vi "Get Boundary and Descriptions.vi"(0 "Image In":T1, 1 "Number of iterations":i32=1, 2 "Out":T1, 3 "In":T1, 5 "Mask In":T1, 9 "Submask":T1, 11 "error in (no error)":errorcluster, 12 "ConvexHull":bool) -> (4 "Boundaries":cluster{cluster{i32, i32}[]}[](array[cluster]), 6 "Reporter":T2(array[cluster]), 10 "Object Descriptions":T3(array[cluster]), 15 "error out":errorcluster)   [LabVIEW 2012, in "Visual Analyser.lvlib"]
uses:
  Visual Analyser.lvlib
  <vilib>/vision/Image Controls.llb/IMAQ Image.ctl
  <vilib>/vision/NI_Vision_Development_Module.lvlib
panel:
  in  "WholeBG %":sgl
  out "#particles":i32
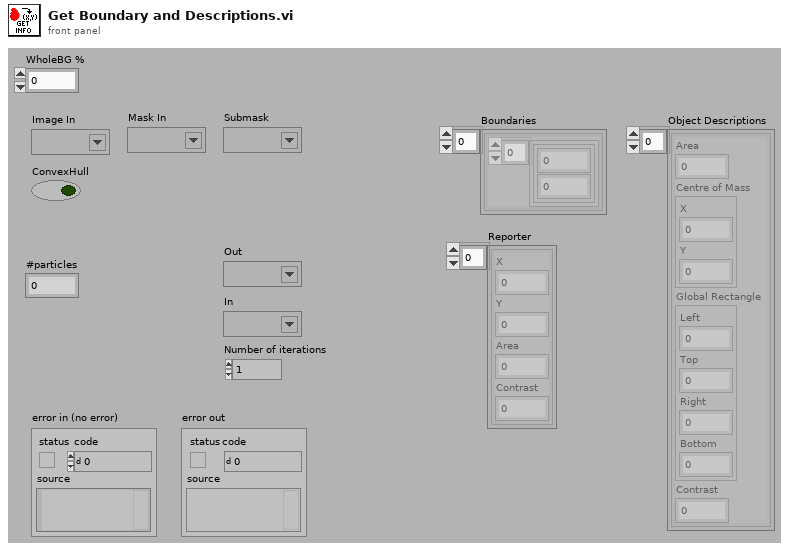
[diagram p1: front panel]
types:
  T1 = typedef "IMAQ Image.ctl" = refnum<image>
  T2 = cluster{"X":dbl, "Y":dbl, "Area":dbl, "Contrast":dbl}[]
  T3 = cluster{"Area":dbl, "Centre of Mass":cluster{"X":dbl, "Y":dbl}, "Global Rectangle":cluster{"Left":dbl, "Top":dbl, "Right":dbl, "Bottom":dbl}, "Contrast":dbl}[]
  T4 = typedef "Particle Parameters" = i32
  T5 = typedef "ROI Descriptor" = cluster{"Global Rectangle":i32[], "Contours":cluster{"ID":enum32{"External", "Internal"}, "Type":u32, "Coordinates":i32[]}[]}
  T6 = enum32{"AutoM", "Close", "Dilate", "Erode", "Gradient", "Gradient out", "Gradient in", "Hit miss", "Open", "PClose", "POpen", "Thick", "Thin"}
  T7 = cluster{"histogram":u32[], "Minimal Value":sgl, "Maximal Value":sgl, "Starting Value":sgl, "Interval Width":sgl, "Mean Value":sgl, "Standard  Variation":sgl, "Area (pixels)":i32}
  T8 = cluster{"ID":enum32{"External", "Internal"}, "Type":u32, "Coordinates":i32[]}[]
  T9 = typedef "IMAQ Rectangle" = cluster{"Left":i32, "Top":i32, "Right":i32, "Bottom":i32, "Rotation":dbl}
  T10 = cluster{"Area":dbl, "Centre of Mass":cluster{"X":dbl, "Y":dbl}, "Global Rectangle":cluster{"Left":dbl, "Top":dbl, "Right":dbl, "Bottom":dbl}, "Contrast":dbl}
  T11 = cluster{"Left":dbl, "Top":dbl, "Right":dbl, "Bottom":dbl}
  T12 = cluster{"X":dbl, "Y":dbl, "Area":dbl, "Contrast":dbl}
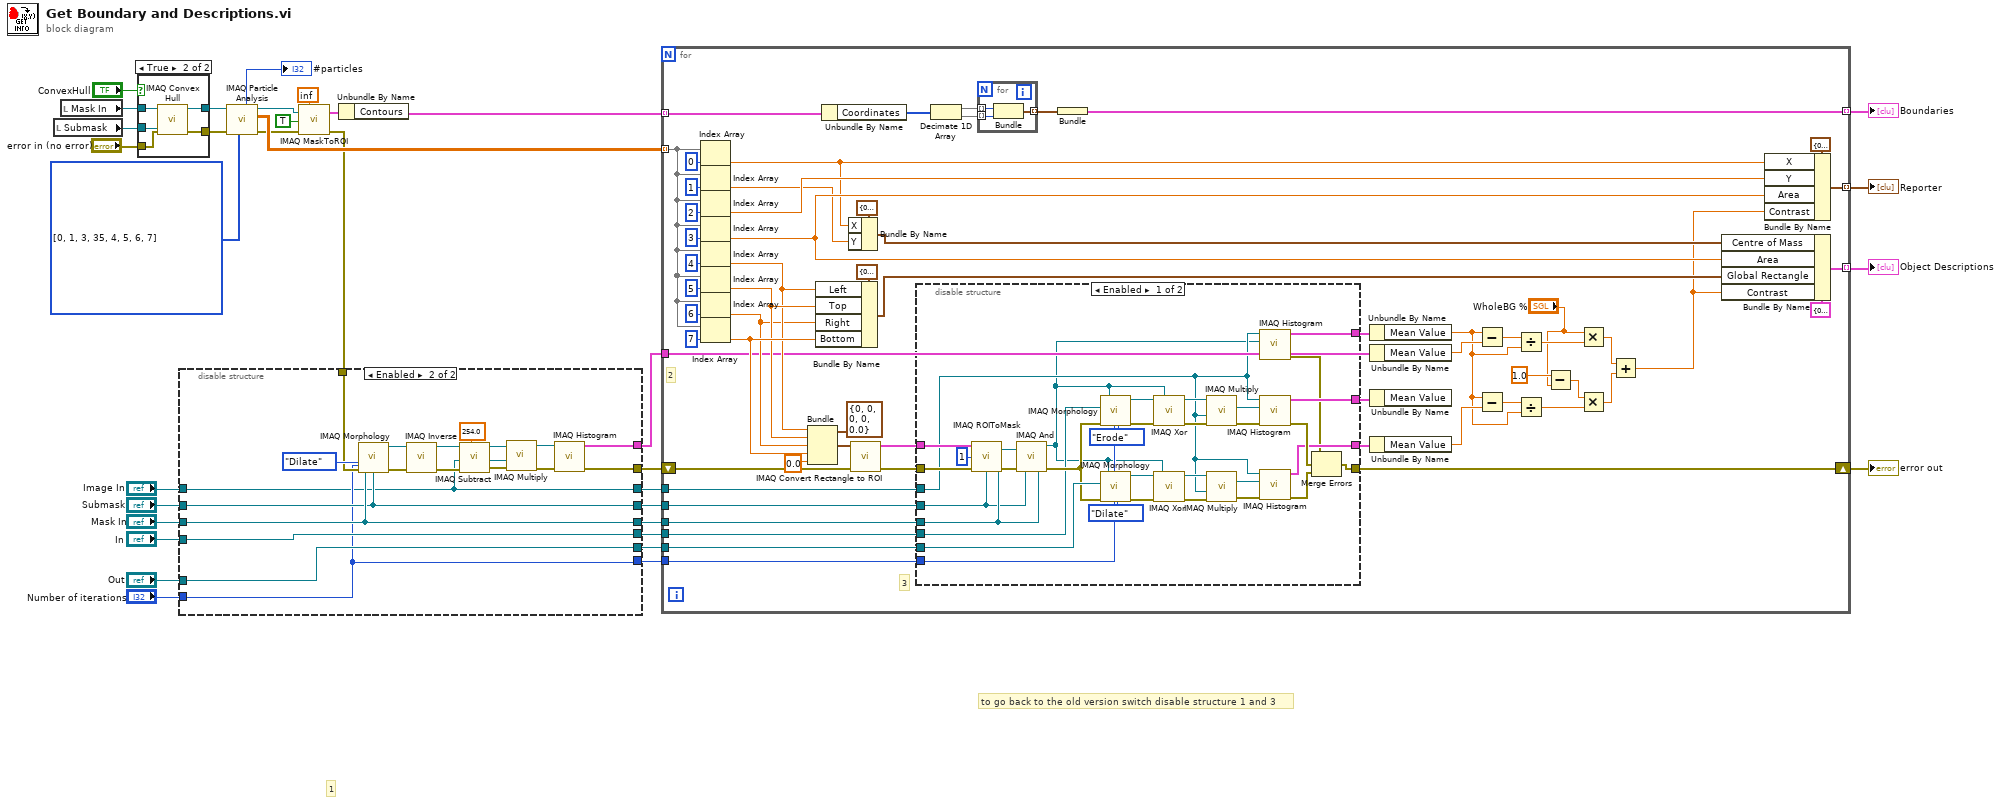
[diagram p0: block diagram]
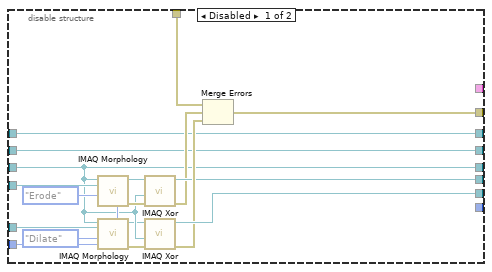
[diagram p2: hidden frame]
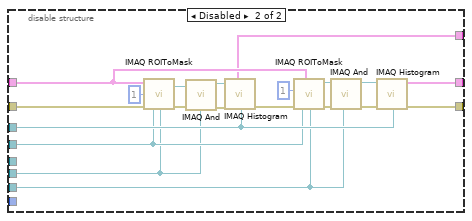
[diagram p4: hidden frame]
diagram:
  w12 = T4[] [0, 1, 3, 35, 4, 5, 6, 7] items=["Center of Mass X", "Center of Mass Y", "First Pixel X", "First Pixel Y", "Bounding Rect Left", "Bounding Rect Top", "Bounding Rect Right", "Bounding Rect Bottom", "Max Feret Diameter Start X", "Max Feret Diameter Start Y", "Max Feret Diameter End X", "Max Feret Diameter End Y", "Max Horiz. Segment Length Left", "Max Horiz. Segment Length Right", "Max Horiz. Segment Length Row", "-", "Bounding Rect Width", "Bounding Rect Height", "Bounding Rect Diagonal", "Perimeter", "Convex Hull Perimeter", "Holes' Perimeter", "Max Feret Diameter", "Equivalent Ellipse Major Axis", "Equivalent Ellipse Minor Axis", "Equivalent Ellipse Minor Axis (Feret)", "Equivalent Rect Long Side", "Equivalent Rect Short Side", "Equivalent Rect Diagonal", "Equivalent Rect Short Side (Feret)", "Average Horiz. Segment Length", "Average Vert. Segment Length", "Hydraulic Radius", "Waddel Disk Diameter", "-", "Area", "Holes' Area", "Particle & Holes' Area", "Convex Hull Area", "Image Area", "-", "Number of Holes", "Number of Horiz. Segments", "Number of Vert. Segments", "-", "Orientation", "Max Feret Diameter Orientation", "-", "% Area/Image Area", "% Area/(Particle & Holes' Area)", "Ratio of Equivalent Ellipse Axes", "Ratio of Equivalent Rect Sides", "-", "Elongation Factor", "Compactness Factor", "Heywood Circularity Factor", "Type Factor", "-", "Sum X", "Sum Y", "Sum XX", "Sum XY", "Sum YY", "Sum XXX", "Sum XXY", "Sum XYY", "Sum YYY", "-", "Moment of Inertia XX", "Moment of Inertia XY", "Moment of Inertia YY", "Moment of Inertia XXX", "Moment of Inertia XXY", "Moment of Inertia XYY", "Moment of Inertia YYY", "Norm. Moment of Inertia XX", "Norm. Moment of Inertia XY", "Norm. Moment of Inertia YY", "Norm. Moment of Inertia XXX", "Norm. Moment of Inertia XXY", "Norm. Moment of Inertia XYY", "Norm. Moment of Inertia YYY", "Hu Moment 1", "Hu Moment 2", "Hu Moment 3", "Hu Moment 4", "Hu Moment 5", "Hu Moment 6", "Hu Moment 7"] ("Pixel Measurements")
  # "1"
  # "to go back to the old version switch disable structure 1 and 3"
  n1 = local read "Submask"() -> (w18:T1)
  n2 = local read "Mask In"() -> (w17:T1)
  n3 = case shown="True" "ConvexHull" {
    tunnel: w18 -> [_ w41]
    tunnel: w17 -> [w36 w40]
    tunnel: [w35 w39] -> w15
    tunnel: [w36 w38] -> w14
    tunnel: "error in (no error)" -> [w35 w37]
    frame False {
    }
    frame True {
      n4 = call "IMAQ Convex Hull"("error in (no error)"=w37, "Image Dst"=w41, "Image Src"=w40) -> ("error out"=w39:errorcluster, "Image Dst Out"=w38:T1)  [unwired: 7 in]
    }
  }
  n5 = call "IMAQ Particle Analysis"("error in (no error)"=w15, "Pixel Measurements"=w12, "Image"=w14) -> ("error out"=w16:errorcluster, "Particle Measurements (Pixels)"=w19:dbl[][], "Image Out (duplicate)"=w13:T1, "Number of Particles"=→"#particles":i32)  [unwired: 2 in, 3 out]
  n6 = call "IMAQ MaskToROI"("External edges only (T)"=TRUE, "Image"=w13, "Max number of vectors in ROI"=inf, "error in (no error)"=w16) -> ("ROI Descriptor"=w20:T5, "error out"=w10:errorcluster)  [unwired: 3 in, 1 out]
  n7 = disable-structure shown="Enabled" {
    disable-tunnel: "In" -> [w54 w78]
    disable-tunnel: "Out" -> [w53 w77]
    disable-tunnel: [w52 w66] -> w28
    disable-tunnel: "Number of iterations" -> [w51 w67]
    disable-tunnel: [w50 w77] -> w26
    disable-tunnel: [w48 w78] -> w25
    disable-tunnel: "Mask In" -> [w43 w74]
    disable-tunnel: w10 -> [w46 w75]
    disable-tunnel: [w43 w74] -> w7
    disable-tunnel: [w44 w73] -> w6
    disable-tunnel: "Submask" -> [w44 w73]
    disable-tunnel: [w45 w63] -> w4
    disable-tunnel: "Image In" -> [w45 w63]
    disable-tunnel: [_ w67] -> w2
    disable-tunnel: [_ w60] -> w1
    frame Disabled {
      n8 = call "IMAQ Morphology"("Number of iterations (1)"=w51, "Operation"=T6."Erode", "Image Dst"=w54, "Image Src"=w43) -> ("error out"=w58:errorcluster, "Image Dst Out"=w59:T1)  [unwired: 6 in]
      n9 = call "IMAQ Morphology"("Number of iterations (1)"=w51, "Operation"=T6."Dilate", "Image Dst"=w53, "Image Src"=w43) -> ("error out"=w57:errorcluster, "Image Dst Out"=w42:T1)  [unwired: 6 in]
      n10 = call "IMAQ Xor"("error in (no error)"=w58, "Image Src B"=w43, "Image Src A"=w59) -> ("error out"=w47:errorcluster, "Image Dst Out"=w48:T1)  [unwired: 7 in]
      n11 = call "IMAQ Xor"("error in (no error)"=w57, "Image Src B"=w43, "Image Src A"=w42) -> ("error out"=w49:errorcluster, "Image Dst Out"=w50:T1)  [unwired: 7 in]
      n12 = Merge Errors(w46, w47, w49) -> (w52:errorcluster)
    }
    frame Enabled {
      n13 = call "IMAQ Morphology"("Number of iterations (1)"=w67, "error in (no error)"=w75, "Operation"=T6."Dilate", "Image Dst"=w73, "Image Src"=w74) -> ("error out"=w72:errorcluster, "Image Dst Out"=w71:T1)  [unwired: 5 in]
      n14 = call "IMAQ Inverse"("error in (no error)"=w72, "Image Src"=w71) -> ("error out"=w70:errorcluster, "Image Dst Out"=w69:T1)  [unwired: 8 in]
      n15 = call "IMAQ Subtract"("Image Src A"=w69, "Constant"=sgl 254.0, "error in (no error)"=w70) -> ("Image Dst Out"=w62:T1, "error out"=w65:errorcluster)  [unwired: 4 in]
      n16 = call "IMAQ Multiply"("Image Src A"=w62, "Image Dst"=w62, "Image Src B"=w63, "error in (no error)"=w65) -> ("Image Dst Out"=w61:T1, "error out"=w64:errorcluster)  [unwired: 3 in]
      n17 = call "IMAQ Histogram"("error in (no error)"=w64, "Image"=w61) -> ("error out"=w66:errorcluster, "Histogram Report"=w60:T7)  [unwired: 8 in]
    }
  }
  n18 = Unbundle By Name(w20) -> ("Contours"=w34:T8)
  n19 = for {
    tunnel: w34 -> [w139] mode=indexing
    tunnel: w7 -> [w102]
    tunnel: w6 -> [w105]
    tunnel: w4 -> [w110]
    tunnel: w19 -> [w119] mode=indexing
    tunnel: [w115] -> w32 mode=indexing
    tunnel: [w118] -> w33 mode=indexing
    tunnel: [w117] -> w31 mode=indexing
    shift-right: [w99] -> w23
    shift-left: w28 -> [w100]
    tunnel: w25 -> [w104]
    tunnel: w26 -> [w103]
    tunnel: w2 -> [w101]
    tunnel: w1 -> [w95]
    # "3"
    # "2"
    n20 = Index Array(array=w119, index=0) -> (element=w109:dbl)
    n21 = Index Array(array=w119, index=1) -> (element=w108:dbl)
    n22 = Index Array(array=w119, index=2) -> (element=w129:dbl)
    n23 = Index Array(array=w119, index=3) -> (element=w135:dbl)
    n24 = Index Array(array=w119, index=4) -> (element=w112:dbl)
    n25 = Index Array(array=w119, index=5) -> (element=w113:dbl)
    n26 = Index Array(array=w119, index=6) -> (element=w111:dbl)
    n27 = Index Array(array=w119, index=7) -> (element=w114:dbl)
    n28 = Bundle(cluster=T9 {"Left"=0, "Top"=0, "Right"=0, "Bottom"=0, "Rotation"=0.0} ("Rectangle"), "Left"=w112, "Top"=w113, "Right"=w111, "Bottom"=w114, "Rotation"=0.0) -> (w93:T9)
    n29 = Bundle By Name(cluster=T11 {"Left"=0.0, "Top"=0.0, "Right"=0.0, "Bottom"=0.0} ("Point Coordinates"), "Left"=w112, "Top"=w113, "Right"=w111, "Bottom"=w114) -> (w132:T11)
    n30 = Unbundle By Name(w139) -> ("Coordinates"=w138:i32[])
    n31 = Bundle By Name(cluster=cluster{"X":dbl, "Y":dbl} {"X"=0.0, "Y"=0.0} ("Point Coordinates"), "X"=w109, "Y"=w108) -> (w134:cluster{"X":dbl, "Y":dbl})
    n32 = call "IMAQ Convert Rectangle to ROI"("error in (no error)"=w100, "Rectangle"=w93) -> ("error out"=w106:errorcluster, "ROI Descriptor"=w107:T5)  [unwired: 7 in]
    n33 = disable-structure shown="Enabled" {
      disable-tunnel: w106 -> [w160 w191]
      disable-tunnel: w105 -> [w170 w179]
      disable-tunnel: w110 -> [w143 w192]
      disable-tunnel: [w147 w193] -> w99
      disable-tunnel: w103 -> [w162 w176]
      disable-tunnel: w104 -> [w157 w177]
      disable-tunnel: w107 -> [w172 w188]
      disable-tunnel: w102 -> [w171 _]
      disable-tunnel: w101 -> [w167 _]
      disable-tunnel: [w146 w175] -> w98
      disable-tunnel: [w145 w174] -> w97
      disable-tunnel: [w144 _] -> w91
      frame Enabled {
        n34 = call "IMAQ ROIToMask"("error in (no error)"=w160, "ROI Descriptor"=w172, "Filling Value (255)"=1, "Image"=w170, "Image Model"=w171) -> ("error out"=w161:errorcluster, "Image Out"=w159:T1)  [unwired: 2 out]
        n35 = call "IMAQ And"("error in (no error)"=w161, "Image Src B"=w171, "Image Dst"=w159, "Image Src A"=w170) -> ("error out"=w158:errorcluster, "Image Dst Out"=w141:T1)  [unwired: 6 in]
        n36 = call "IMAQ Morphology"("Number of iterations (1)"=w167, "error in (no error)"=w158, "Operation"=T6."Erode", "Image Dst"=w157, "Image Src"=w141) -> ("error out"=w165:errorcluster, "Image Dst Out"=w166:T1)  [unwired: 5 in]
        n37 = call "IMAQ Morphology"("Number of iterations (1)"=w167, "error in (no error)"=w158, "Operation"=T6."Dilate", "Image Dst"=w162, "Image Src"=w141) -> ("error out"=w163:errorcluster, "Image Dst Out"=w164:T1)  [unwired: 5 in]
        n38 = call "IMAQ Xor"("error in (no error)"=w165, "Image Src B"=w141, "Image Src A"=w166) -> ("error out"=w156:errorcluster, "Image Dst Out"=w153:T1)  [unwired: 7 in]
        n39 = call "IMAQ Xor"("error in (no error)"=w163, "Image Src B"=w141, "Image Src A"=w164) -> ("error out"=w155:errorcluster, "Image Dst Out"=w154:T1)  [unwired: 7 in]
        n40 = call "IMAQ Multiply"("Image Src A"=w153, "Image Src B"=w143, "error in (no error)"=w156) -> ("Image Dst Out"=w150:T1, "error out"=w152:errorcluster)  [unwired: 4 in]
        n41 = call "IMAQ Multiply"("Image Src A"=w154, "Image Src B"=w143, "error in (no error)"=w155) -> ("Image Dst Out"=w140:T1, "error out"=w151:errorcluster)  [unwired: 4 in]
        n42 = call "IMAQ Histogram"("Image Mask"=w141, "Image"=w143) -> ("error out"=w142:errorcluster, "Histogram Report"=w144:T7)  [unwired: 8 in]
        n43 = call "IMAQ Histogram"("error in (no error)"=w152, "Image Mask"=w150, "Image"=w143) -> ("error out"=w149:errorcluster, "Histogram Report"=w145:T7)  [unwired: 7 in]
        n44 = call "IMAQ Histogram"("error in (no error)"=w151, "Image Mask"=w140, "Image"=w143) -> ("error out"=w148:errorcluster, "Histogram Report"=w146:T7)  [unwired: 7 in]
        n45 = Merge Errors(w142, w149, w148) -> (w147:errorcluster)
      }
      frame Disabled {
        n46 = call "IMAQ ROIToMask"("error in (no error)"=w191, "ROI Descriptor"=w188, "Filling Value (255)"=1, "Image"=w179, "Image Model"=w177) -> ("error out"=w187:errorcluster, "Image Out"=w183:T1)  [unwired: 2 out]
        n47 = call "IMAQ And"("error in (no error)"=w187, "Image Src B"=w177, "Image Src A"=w183) -> ("error out"=w186:errorcluster, "Image Dst Out"=w181:T1)  [unwired: 7 in]
        n48 = call "IMAQ Histogram"("error in (no error)"=w186, "Image Mask"=w181, "Image"=w192) -> ("error out"=w189:errorcluster, "Histogram Report"=w174:T7)  [unwired: 7 in]
        n49 = call "IMAQ ROIToMask"("error in (no error)"=w189, "ROI Descriptor"=w188, "Filling Value (255)"=1, "Image"=w179, "Image Model"=w176) -> ("error out"=w184:errorcluster, "Image Out"=w182:T1)  [unwired: 2 out]
        n50 = call "IMAQ And"("error in (no error)"=w184, "Image Src B"=w176, "Image Src A"=w182) -> ("error out"=w185:errorcluster, "Image Dst Out"=w180:T1)  [unwired: 7 in]
        n51 = call "IMAQ Histogram"("error in (no error)"=w185, "Image Mask"=w180, "Image"=w192) -> ("error out"=w193:errorcluster, "Histogram Report"=w175:T7)  [unwired: 7 in]
      }
    }
    n52 = Decimate 1D Array(w138) -> (w137:i32[], w136:i32[])
    n53 = for {
      tunnel: w137 -> [w196] mode=indexing
      tunnel: w136 -> [w195] mode=indexing
      tunnel: [w194] -> w116 mode=indexing
      n54 = Bundle(w196, w195) -> (w194:cluster{i32, i32})  [unwired: 1 in]
    }
    n55 = Bundle(w116) -> (w115:cluster{cluster{i32, i32}[]})  [unwired: 1 in]
    n56 = Unbundle By Name(w91) -> ("Mean Value"=w79:sgl)
    n57 = Unbundle By Name(w95) -> ("Mean Value"=w90:sgl)
    n58 = Unbundle By Name(w97) -> ()  [unwired: 1 out]
    n59 = Unbundle By Name(w98) -> ("Mean Value"=w88:sgl)
    n60 = Subtract(x=w79, y=w90) -> (x-y=w89:sgl)
    n61 = Subtract(x=w79, y=w88) -> (x-y=w96:sgl)
    n62 = Divide(x=w89, y=w79) -> (x/y=w87:sgl)
    n63 = Divide(x=w96, y=w79) -> (x/y=w86:sgl)
    n64 = Subtract(x=1.0, y="WholeBG %") -> (x-y=w84:dbl)
    n65 = Multiply(x="WholeBG %", y=w87) -> (x*y=w83:sgl)
    n66 = Multiply(x=w84, y=w86) -> (x*y=w82:dbl)
    n67 = Add(x=w83, y=w82) -> (x+y=w81:dbl)
    n68 = Bundle By Name(cluster=T10 {"Area"=0.0, "Centre of Mass"={"X"=0.0, "Y"=0.0}, "Global Rectangle"={"Left"=0.0, "Top"=0.0, "Right"=0.0, "Bottom"=0.0}, "Contrast"=0.0}, "Centre of Mass"=w134, "Area"=w135, "Global Rectangle"=w132, "Contrast"=w81) -> (w118:T10)
    n69 = Bundle By Name(cluster=T12 {"X"=0.0, "Y"=0.0, "Area"=0.0, "Contrast"=0.0} ("Point Coordinates"), "X"=w109, "Y"=w129, "Area"=w135, "Contrast"=w81) -> (w117:T12)
  }
  "error out" <- w23
  "Object Descriptions" <- w33
  "Boundaries" <- w32
  "Reporter" <- w31
